vi "SolenoidSet_Double_InverSingle.vi"(1 "Solenoid 2":string, 2 "Solenoid 1 (Inverted)":string, 3 "Switch To":bool) -> ()   [LabVIEW 2016]
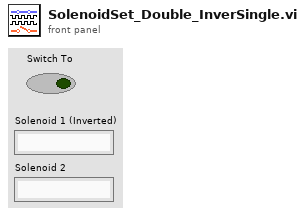
[diagram p1: front panel]
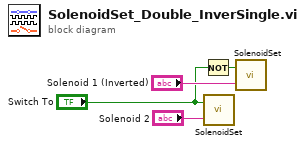
[diagram p0: block diagram]
diagram:
  n1 = Not(x="Switch To") -> (.not. x?=w1:bool)
  n2 = call "SolenoidSet.vi"("String"="Solenoid 2", "Boolean"="Switch To") -> ()
  n3 = call "SolenoidSet.vi"("String"="Solenoid 1 (Inverted)", "Boolean"=w1) -> ()
